vi "Vision Processing.vi"(4 "error in (no error)":errorcluster, 7 "Image Size":T2) -> ()   [LabVIEW 2015]
doc: "This VI runs in parallel to other tasks. It gets images from the camera, processes them for color or shape and use that information to affect robot behavior."
uses:
  <vilib>/Rock Robotics/WPI/Camera/WPI_CameraImageSize.ctl
  <vilib>/Rock Robotics/WPI/Camera/WPI_CameraExposure Values.ctl
  <vilib>/Rock Robotics/WPI/Camera/WPI_CameraFrameRate.ctl
  Robot Global Data.vi
  Utilities/VisionGlobals.vi
  <vilib>/Rock Robotics/WPI/Camera/WPI_CameraWhite Balance Values.ctl
panel:
  out "Image":T1(plugin-control)
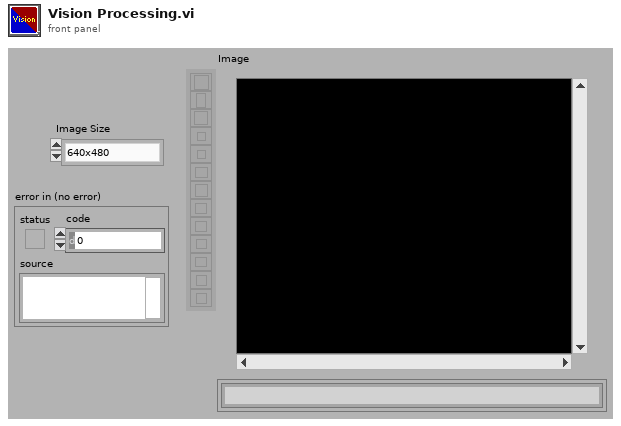
[diagram p1: front panel]
types:
  T1 = typedef "IMAQ Image.ctl" = refnum<image>
  T2 = typedef "WPI_CameraImageSize.ctl" = enum16{"640x480", "320x240", "160x120", "Custom"}
  T3 = typedef "WPI_CameraFrameRate.ctl" = u32
  T4 = typedef "WPI_CameraExposure Values.ctl" = enum16{"Auto", "Flicker-free 50 Hz", "Flicker-free 60 Hz", "Hold current", "Custom"}
  T5 = typedef "Image Type" = u32
  T6 = typedef "WPI_CameraDevRef.ctl" = cluster{"Camera Address":string, "CameraStatus":errorcluster}
  T7 = typedef "WPI_CameraWhite Balance Values.ctl" = enum16{"Auto", "Fixed indoor", "Fixed outdoor 1", "Fixed outdoor 2", "Fixed fluorescent 1", "Fixed fluorescent 2", "Hold current", "Custom"}
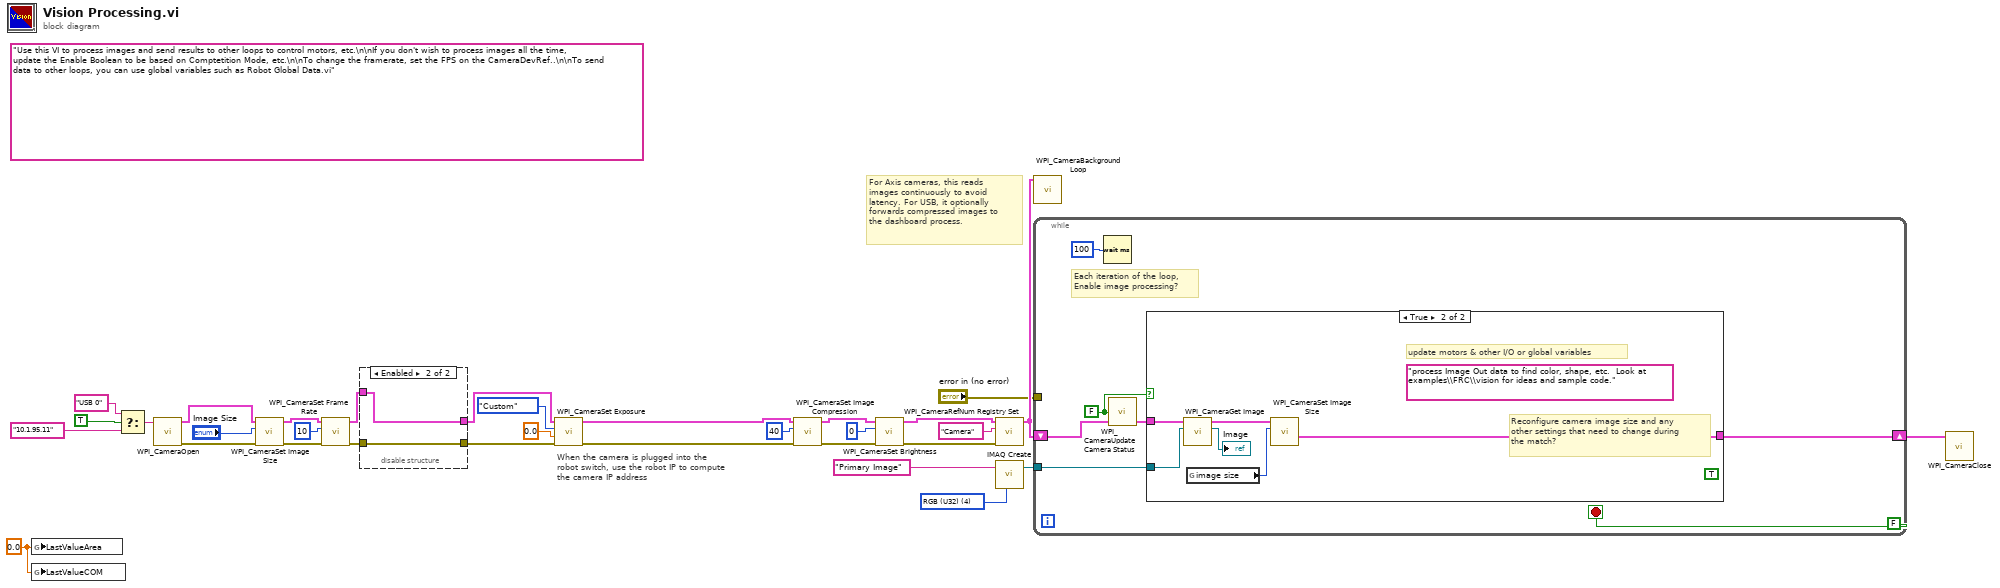
[diagram p0: block diagram]
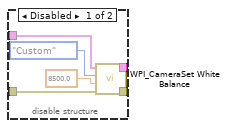
[diagram p2: hidden frame]
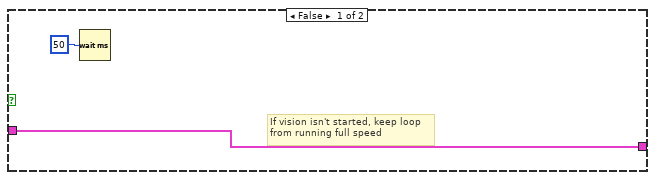
[diagram p3: hidden frame]
diagram:
  w1 = 0.0 ("LastValueArea")
  (unwired) "Use this VI to process images and send results to other loops to control motors, etc.\n\nIf you don't wish to process images all the time, update the Enable Boolean to be based on Comptetition Mode, etc.\n\nTo change the framerate, set the FPS on the CameraDevRef..\n\nTo send data to other loops, you can use global variables such as Robot Global Data.vi"
  w32 = T5 4 items=["Grayscale (U8)", "Grayscale (I16)", "Grayscale (SGL)", "Complex (CSG)", "RGB (U32)", "HSL (U32)", "RGB (U64)"] ("Image Type")
  # "When the camera is plugged into the\nrobot switch, use the robot IP to compute\nthe camera IP address"
  # "For Axis cameras, this reads\nimages continuously to avoid\nlatency. For USB, it optionally\nforwards compressed images to\nthe dashboard process."
  n1 = global write "VisionGlobals.vi" "LastValueArea"(w1) -> ()
  n2 = global write "VisionGlobals.vi" "LastValueCOM"(w1) -> ()
  n3 = Select(t="USB 0" ("format string"), s=TRUE ("dot notation? (F)"), f="10.1.95.11" ("format string")) -> (s? t:f=w4:string)
  n4 = call <vilib>:"WPI_CameraOpen.vi"("Camera Address"=w4) -> ("error out"=w20:errorcluster, "CameraDevRef"=w21:T6)  [unwired: 1 in, 8 out]
  n5 = call <vilib>:"WPI_CameraSet Image Size.vi"("error in (no error)"=w20, "Image Size"="Image Size", "CameraDevRef"=w21) -> ("error out"=w19:errorcluster, "CameraDevRef Out"=w22:T6)  [unwired: 1 in, 6 out]
  n6 = call <vilib>:"WPI_CameraSet Frame Rate.vi"("error in (no error)"=w19, "Frame Rate (fps)"=T3 10, "CameraDevRef"=w22) -> ("error out"=w18:errorcluster, "CameraDevRef Out"=w24:T6)  [unwired: 7 out]
  n7 = disable-structure shown="Enabled" {
    disable-tunnel: w24 -> [w38 w40]
    disable-tunnel: [w37 w40] -> w23
    disable-tunnel: w18 -> [w36 w39]
    disable-tunnel: [w35 w39] -> w17
    frame Disabled {
      n8 = call <vilib>:"WPI_CameraSet White Balance.vi"("error in (no error)"=w36, "Color Temp (K)"=8500.0, "White Balance"=WPI_CameraWhite_Balance_Values."Custom", "CameraDevRef"=w38) -> ("error out"=w35:errorcluster, "CameraDevRef Out"=w37:T6)  [unwired: 6 out]
    }
    frame Enabled {
    }
  }
  n9 = call <vilib>:"WPI_CameraSet Exposure.vi"("error in (no error)"=w17, "Exposure (%)"=0.0, "Exposure"=WPI_CameraExposure_Values."Custom", "CameraDevRef"=w23) -> ("error out"=w16:errorcluster, "CameraDevRef Out"=w26:T6)  [unwired: 6 out]
  n10 = call <vilib>:"WPI_CameraSet Image Compression.vi"("error in (no error)"=w16, "Compression"=40, "CameraDevRef"=w26) -> ("error out"=w15:errorcluster, "CameraDevRef Out"=w25:T6)  [unwired: 7 out]
  n11 = call <vilib>:"WPI_CameraSet Brightness.vi"("error in (no error)"=w15, "Brightness"=0, "CameraDevRef"=w25) -> ("error out"=w13:errorcluster, "CameraDevRef Out"=w14:T6)  [unwired: 7 out]
  n12 = call <vilib>:"WPI_CameraRefNum Registry Set.vi"("error in (no error)"=w13, "refnum name"="Camera", "CameraDevRef"=w14) -> ("CameraDevRef"=w10:T6)  [unwired: 1 in, 7 out]
  n13 = call "IMAQ Create"("Image Name"="Primary Image", "Image Type"=w32) -> ("New Image"=w30:T1)  [unwired: 2 in, 2 out]
  n14 = call <vilib>:"WPI_CameraBackground Loop.vi"("CameraDevRef"=w10) -> ()  [unwired: 11 in]
  n15 = while {
    shift-right: [w46] -> w8
    shift-left: w10 -> [w44]
    tunnel: w30 -> [w45]
    tunnel: "error in (no error)" -> [_]
    stop <- FALSE stop-if-true
    w41 = FALSE ("Enable Vision")
    # "Each iteration of the loop,\nEnable image processing?"
    n16 = Wait (ms)(milliseconds to wait=u32 100) -> ()  [unwired: 1 out]
    n17 = call <vilib>:"WPI_CameraUpdate Camera Status.vi"("CameraDevRef In"=w44, "Enable Vision"=w41) -> ("CameraDevRef Out"=w43:T6)  [unwired: 3 in]
    n18 = case shown="True" w41 {
      tunnel: w45 -> [_ w54]
      tunnel: [w49 w55] -> w46
      tunnel: w43 -> [w49 w52]
      frame False {
        # "If vision isn't started, keep loop\nfrom running full speed"
        n19 = Wait (ms)(milliseconds to wait=u32 50) -> ()  [unwired: 1 out]
      }
      frame True {
        (unwired) TRUE
        (unwired) "process Image Out data to find color, shape, etc.  Look at examples\\FRC\\vision for ideas and sample code."
        # "update motors & other I/O or global variables"
        # "Reconfigure camera image size and any\nother settings that need to change during\nthe match?"
        n20 = call <vilib>:"WPI_CameraGet Image.vi"("Image"=w54, "CameraDevRef"=w52) -> ("Image Out"=→"Image":T1, "CameraDevRef Out"=w51:T6)  [unwired: 1 in, 7 out]
        n21 = global read "Robot Global Data.vi" "image size"() -> (w53:T2)
        n22 = call <vilib>:"WPI_CameraSet Image Size.vi"("Image Size"=w53, "CameraDevRef"=w51) -> ("CameraDevRef Out"=w55:T6)  [unwired: 2 in, 7 out]
      }
    }
  }
  n23 = call <vilib>:"WPI_CameraClose.vi"("CameraDevRef"=w8) -> ()  [unwired: 1 in, 10 out]
